vi "Split Data for Crossvalidation.vi"() -> ()   [LabVIEW 2016]
uses:
  _XML_EEG_Features/XML_FF_Trial.ctl
  _vlib/ClassifierClass.lvclass
  Classifier.lvlib
  _XML_EEG_Features/XML_EEG_Features.lvlib
panel:
  in  "Number of Folds":i32=5 caption="Число раундов кросс-проверки" min=5 max=100 step=1
  out "Number of Trials of each Class":i32[](array[numeric]) caption="Число проб каждого класса"
  out "AppState":string caption="Состояние"
  in  "Start":bool
  in  "Stop":bool
  out "Progress":i32(slide) caption="Ход выполнения" scale=0.0..10.0
  in  "Path To XML File":path caption="Путь к XML файлу"
  out "CLassLabels out":string[](array[string]) caption="Метки классов"
  out "EEG Feature Vectors":T1[](array[typedef]) caption="Пробы, загруженные из файла"
  # "This VI is a part of BCI Design library, http://www.ru-bci.org \nCopyright © 2020, Sotnikov Peter, All rights reserved. License: GNU GPLv3"
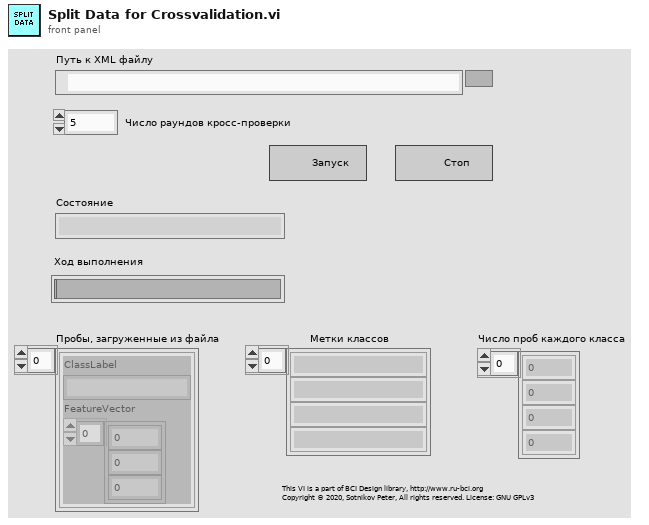
[diagram p1: front panel]
types:
  T1 = typedef "XML_EEG_Features.lvlib/XML_FF_Trial.ctl" = cluster{"ClassLabel":string, "FeatureVector":dbl[]}
  T2 = enum16{"Initialize", "Reading Data", "Split Data To Subsets", "Stop"}
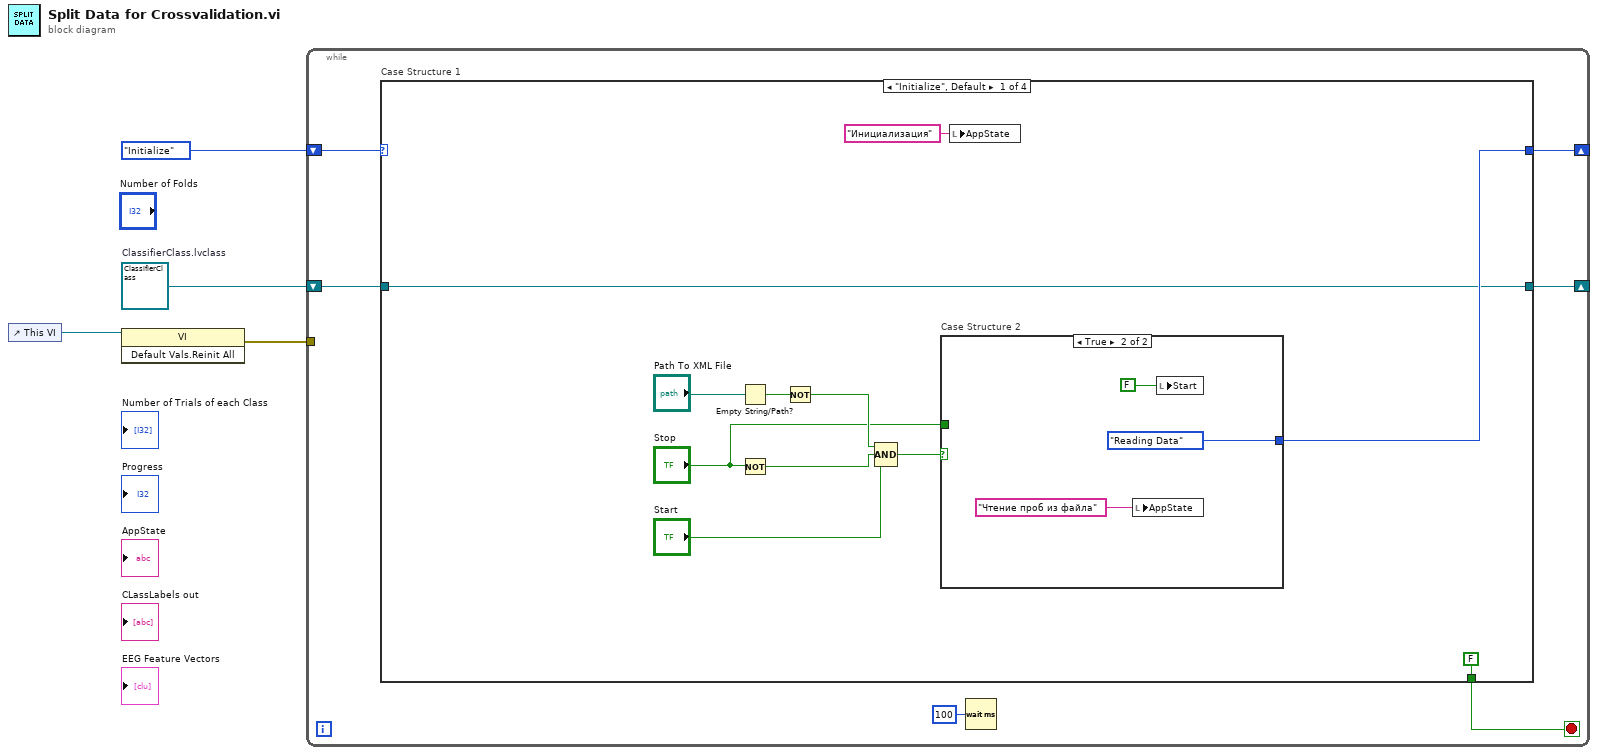
[diagram p0: block diagram]
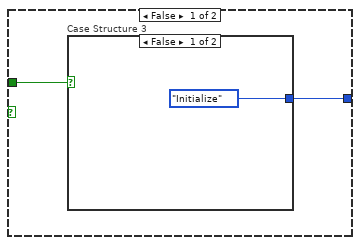
[diagram p2: hidden frame]
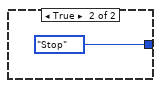
[diagram p3: hidden frame]
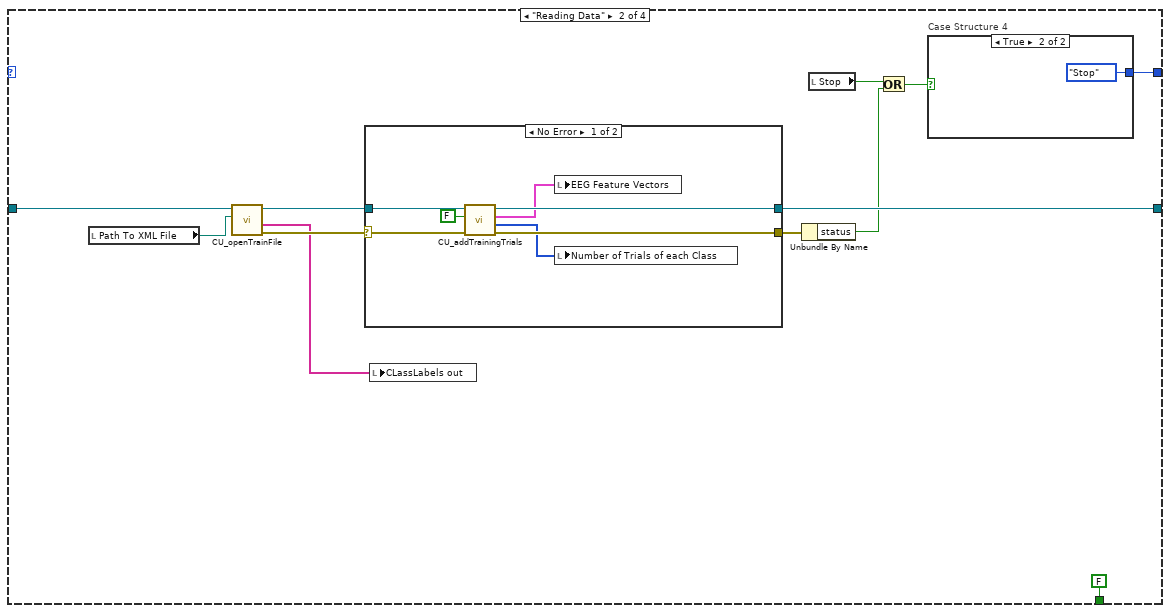
[diagram p4: hidden frame]
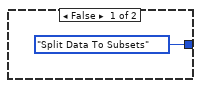
[diagram p6: hidden frame]
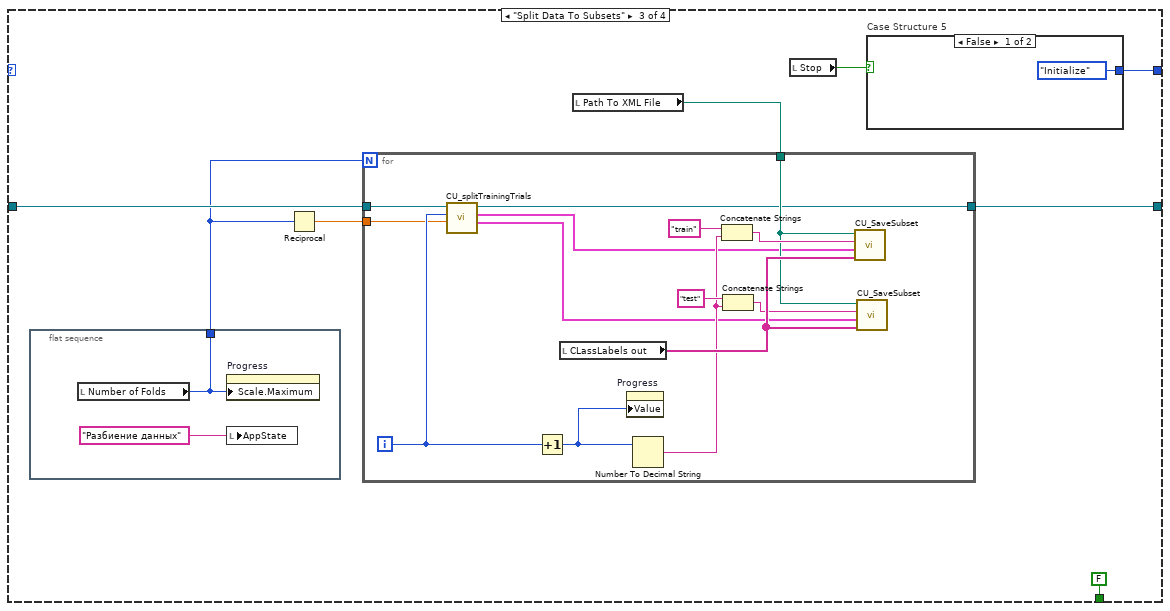
[diagram p7: hidden frame]
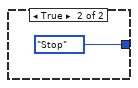
[diagram p8: hidden frame]
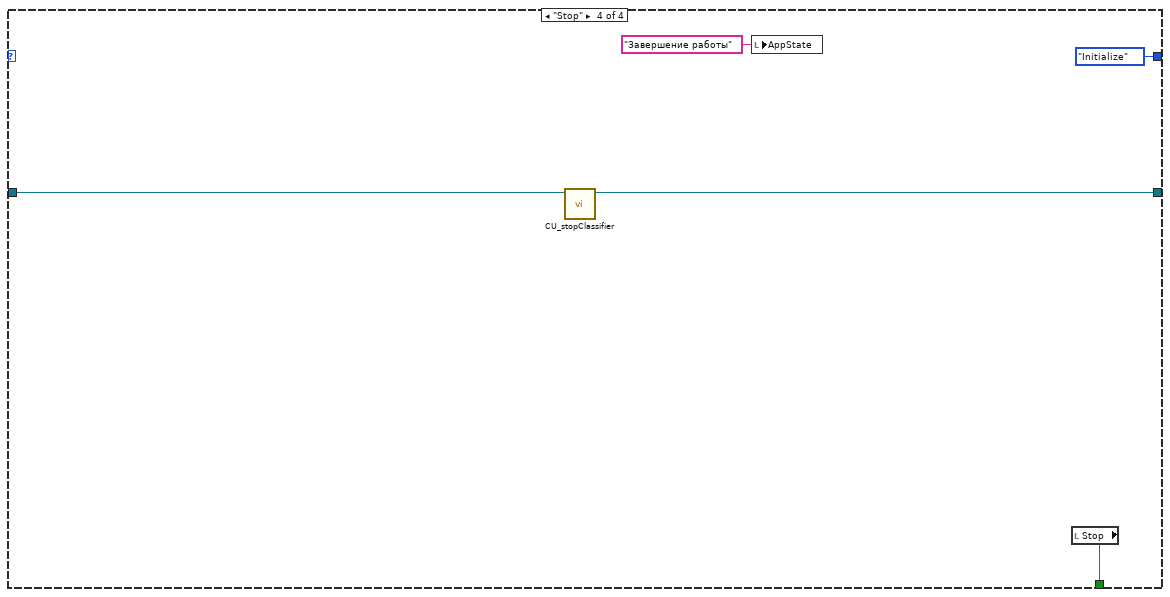
[diagram p9: hidden frame]
diagram:
  w1 = refnum<class "ClassifierClass.lvclass"> refnum  # ClassifierClass.lvclass
  n1 = control-ref of="This VI"() -> (w3:refnum<vi>)
  n2 = invoke class="VI" method="Default Vals.Reinit All"(reference=w3) -> (error out=w2:errorcluster)  [unwired: 2 in, 2 out]
  n3 = while {
    shift-right: [w9] -> _
    shift-left: T2."Initialize" -> [w10]
    tunnel: w2 -> [_]
    shift-right: [w5] -> _
    shift-left: w1 -> [w6]
    stop <- w8 stop-if-true
    n4 = case "Case Structure 1" shown="\"Initialize\", Default" w10 {
      tunnel: [w21 w40 w59 T2."Initialize"] -> w9
      tunnel: [FALSE FALSE FALSE w78] -> w8
      tunnel: w6 -> [w11 w38 w55 w80]
      tunnel: [w11 w34 w54 w79] -> w5
      frame "Initialize", Default {
        n5 = Empty String/Path?(string/path="Path To XML File") -> (empty?=w19:bool)
        n6 = Not(x="Stop") -> (.not. x?=w17:bool)
        n7 = Not(x=w19) -> (.not. x?=w18:bool)
        n8 = Compound Arithmetic op=AND(w18, w17, "Start") -> (w15:bool)
        n9 = case "Case Structure 2" shown="True" w15 {
          tunnel: [w22 T2."Reading Data"] -> w21
          tunnel: "Stop" -> [w23 _]
          frame False {
            n10 = case "Case Structure 3" shown="False" w23 {
              tunnel: [T2."Initialize" T2."Stop"] -> w22
              frame False {
              }
              frame True {
              }
            }
          }
          frame True {
            n11 = local write "AppState"("Чтение проб из файла" ("AppState")) -> ()
            n12 = local write "Start"(FALSE ("Start")) -> ()
          }
        }
        n13 = local write "AppState"("Инициализация" ("AppState")) -> ()
      }
      frame "Reading Data" {
        n14 = local read "Path To XML File"() -> (w35:path)
        n15 = call "CU_openTrainFile.vi"("Path to XML file in"=w35, "ClassifierClass in"=w38) -> ("error out"=w36:errorcluster, "CLass Labels out"=w33:string[], "ClassifierClass out"=w37:refnum<class "ClassifierClass.lvclass">)  [unwired: 6 in, 1 out]
        n16 = case shown="No Error" w36 {
          selector: w36 -> [w44 w48]
          tunnel: w37 -> [w47 w49]
          tunnel: [w45 w49] -> w34
          tunnel: [w43 w48] -> w32
          frame No Error {
            n17 = call "CU_addTrainingTrials.vi"("error in (no error)"=w44, "Use equal number of trials?"=FALSE, "ClassifierClass in"=w47) -> ("error out"=w43:errorcluster, "Num of Trials of each Class"=w42:i32[], "Array of Training Trials out"=w41:T1[], "ClassifierClass out"=w45:refnum<class "ClassifierClass.lvclass">)  [unwired: 5 in]
            n18 = local write "EEG Feature Vectors"(w41) -> ()
            n19 = local write "Number of Trials of each Class"(w42) -> ()
          }
          frame Error {
          }
        }
        n20 = local write "CLassLabels out"(w33) -> ()
        n21 = Unbundle By Name(w32) -> ("status"=w30:bool)
        n22 = local read "Stop"() -> (w31:bool)
        n23 = Or(x=w31, y=w30) -> (x .or. y?=w29:bool)
        n24 = case "Case Structure 4" shown="True" w29 {
          tunnel: [T2."Split Data To Subsets" T2."Stop"] -> w40
          frame False {
          }
          frame True {
          }
        }
      }
      frame "Split Data To Subsets" {
        n25 = flat-sequence {
          tunnel: [w60] -> w53
          frame #0 {
            n26 = local read "Number of Folds"() -> (w60:i32)
            n27 = property on="Progress" class="Slide (strict)"("Scale.Maximum"=w60) -> ()  [unwired: 2 in, 2 out]
            n28 = local write "AppState"("Разбиение данных" ("AppState")) -> ()
          }
        }
        n29 = Reciprocal(x=w53) -> (1/x=w52:dbl)
        n30 = local read "Path To XML File"() -> (w56:path)
        n31 = for {
          N: w53 -> [_]
          tunnel: w56 -> [w71]
          tunnel: w55 -> [w69]
          tunnel: [w68] -> w54
          tunnel: w52 -> [w64]
          i -> [w65]
          n32 = call "CU_splitTrainingTrials.vi"("Portion of test data"=w64, "Iteration"=w65, "ClassifierClass in"=w69) -> ("Array of Check Trials out"=w67:T1[], "Array of Training Trials out"=w66:T1[], "ClassifierClass out"=w68:refnum<class "ClassifierClass.lvclass">)  [unwired: 5 in, 1 out]
          n33 = Increment(x=w65) -> (x+1=w70:i32)
          n34 = local read "CLassLabels out"() -> (w77:string[])
          n35 = property on="Progress" class="Slide (strict)"("Value"=w70) -> ()  [unwired: 2 in, 2 out]
          n36 = Number To Decimal String(number=w70) -> (decimal integer string=w72:string)  [unwired: 1 in]
          n37 = Concatenate Strings("train" ("string"), w72) -> (w76:string)
          n38 = Concatenate Strings("test" ("string"), w72) -> (w75:string)
          n39 = call "CU_SaveSubset.vi"("CLassLabels"=w77, "EEG Feature Vectors"=w66, "Suffix"=w76, "XML file path"=w71) -> ()  [unwired: 7 in, 1 out]
          n40 = call "CU_SaveSubset.vi"("CLassLabels"=w77, "EEG Feature Vectors"=w67, "Suffix"=w75, "XML file path"=w71) -> ()  [unwired: 7 in, 1 out]
        }
        n41 = local read "Stop"() -> (w58:bool)
        n42 = case "Case Structure 5" shown="False" w58 {
          tunnel: [T2."Initialize" T2."Stop"] -> w59
          frame False {
          }
          frame True {
          }
        }
      }
      frame "Stop" {
        n43 = call "CU_stopClassifier.vi"("ClassifierClass in"=w80) -> ("ClassifierClass out"=w79:refnum<class "ClassifierClass.lvclass">)  [unwired: 9 in, 1 out]
        n44 = local write "AppState"("Завершение работы" ("AppState")) -> ()
        n45 = local read "Stop"() -> (w78:bool)
      }
    }
    n46 = Wait (ms)(milliseconds to wait=u32 100) -> ()  [unwired: 1 out]
  }
